vi "ROI_to_bbox.vi"(8 "Image path":path=path "C:/Users/Naomi Tan/Documents/Gillette/ML/STIR_ML_dev/LabView/original_images/IMG_6155.JPG", 9 "Bounding box size":dbl=300.0, 10 "ROI":T5, 11 "Image in":T1) -> (3 "bbox":T2)   [LabVIEW 2024]
uses:
  <vilib>/vision/Image Controls.llb/IMAQ Image.ctl
  controls/class.ctl
panel:
  out "Points":i32[](array[numeric])
  in  "Class Name:":T3 items=["nick", "hair", "cut"]
  out "Classes":string[][](array[string])
  in  "Init Classes":string[][](array[string])
  in  "Size":i32
  out "Bounding Boxes Out":T4(array[cluster])
  in  "Bounding Boxes In":T4(array[cluster])
  in  "Image In":T1
  out "Image Out":T1
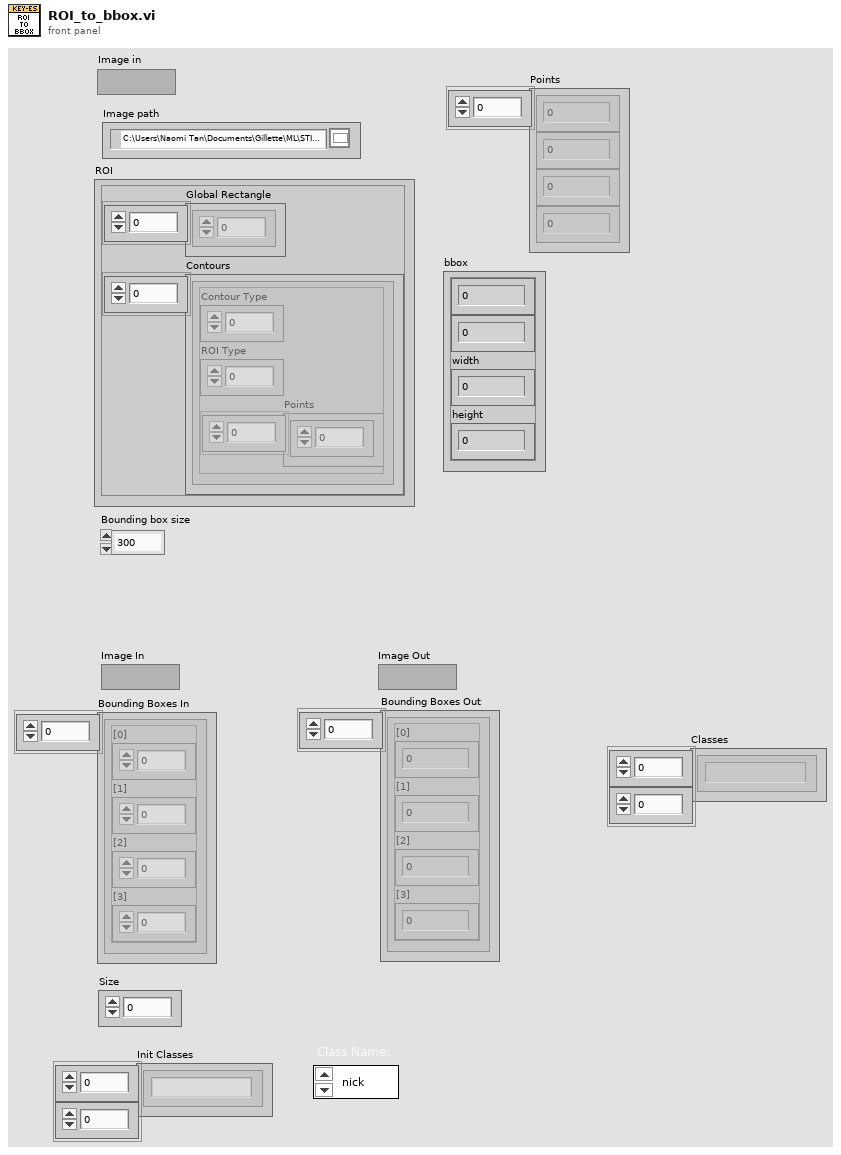
[diagram p1: front panel]
types:
  T1 = typedef "IMAQ Image.ctl" = refnum<image>
  T2 = cluster{"Numeric Control":dbl, "Numeric Control":dbl, "width":dbl, "height":dbl}
  T3 = typedef "Class.ctl" = u16
  T4 = cluster{"[0]":i32, "[1]":i32, "[2]":i32, "[3]":i32}[]
  T5 = cluster{"Global Rectangle":i32[], "Contours":cluster{"Contour Type":u32, "ROI Type":u32, "Points":i32[]}[]}
  T6 = cluster{"Contour Type":u32, "ROI Type":u32, "Points":i32[]}[]
  T7 = cluster{"Contour Type":u32, "ROI Type":u32, "Points":i32[]}
  T8 = typedef "imagedata.ctl" = cluster{"image type":i32, "image depth":i32, "image":u8[], "mask":u8[], "colors":u32[], "Rectangle":cluster{"left":i16, "top":i16, "right":i16, "bottom":i16}}
  T9 = cluster{dbl, dbl, "X Resolution":dbl, "Y Resolution":dbl}
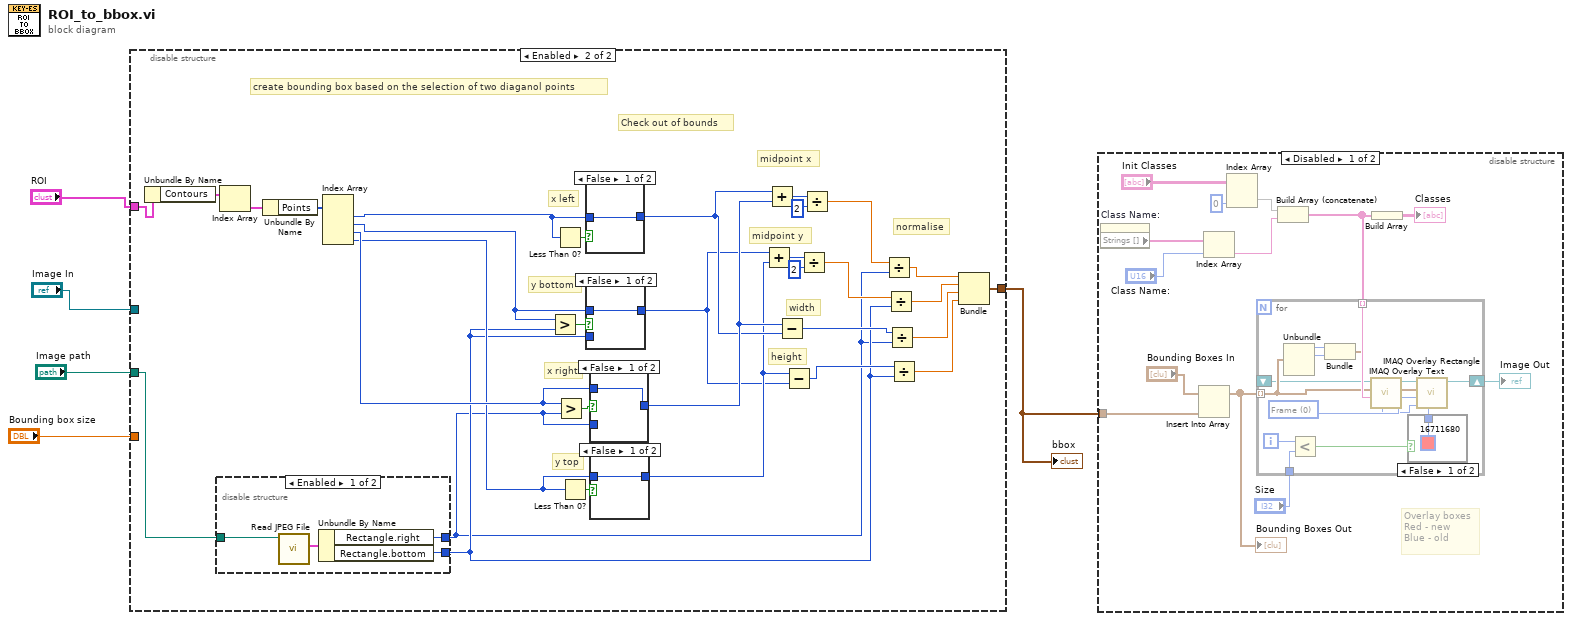
[diagram p0: block diagram]
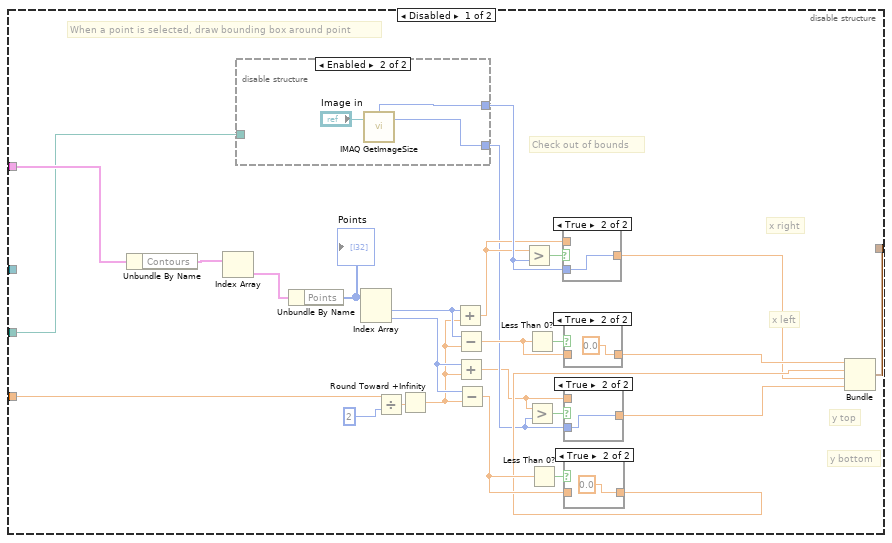
[diagram p2: hidden frame]
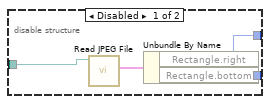
[diagram p3: hidden frame]
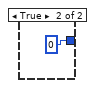
[diagram p8: hidden frame]
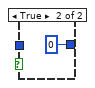
[diagram p11: hidden frame]
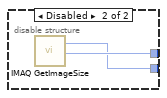
[diagram p12: hidden frame]
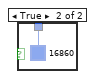
[diagram p13: hidden frame]
diagram:
  n1 = disable-structure shown="Enabled" {
    disable-tunnel: "ROI" -> [w9 w74]
    disable-tunnel: [w8 w71] -> w5
    disable-tunnel: "Bounding box size" -> [w7 _]
    disable-tunnel: "Image In" -> [_ _]
    disable-tunnel: "Image path" -> [w6 w69]
    frame Disabled {
      # "y bottom"
      # "y top"
      # "x left"
      # "x right"
      # "Check out of bounds"
      # "When a point is selected, draw bounding box around point"
      n2 = Unbundle By Name(w9) -> ("Contours"=w31:T6)
      n3 = Index Array(array=w31) -> (element=w30:T7)  [unwired: 1 in]
      n4 = disable-structure shown="Enabled" {
        disable-tunnel: [w34 w38] -> w16
        disable-tunnel: [w33 w37] -> w12
        disable-tunnel: w6 -> [w32 _]
        frame Disabled {
          n5 = call <vilib>:"Read JPEG File.vi"("path to JPEG file"=w32) -> ("image data"=w35:T8)  [unwired: 8 in, 2 out]
          n6 = Unbundle By Name(w35) -> ("Rectangle.right"=w34:i16, "Rectangle.bottom"=w33:i16)
        }
        frame Enabled {
          n7 = call "IMAQ GetImageSize"("Image"="Image in") -> ("Y Resolution"=w37:i32, "X Resolution"=w38:i32)  [unwired: 3 in, 1 out]
        }
      }
      n8 = Unbundle By Name(w30) -> ("Points"=w29:i32[])
      "Points" <- w29
      n9 = Index Array(array=w29) -> (element #1=w27:i32, element #2=w28:i32)  [unwired: 2 in]
      n10 = Divide(x=w7, y=2) -> (x/y=w25:dbl)
      n11 = Round Toward +Infinity(x=w25) -> (ceil(x): smallest int >= x=w24:dbl)
      n12 = Add(x=w27, y=w24) -> (x+y=w15:dbl)
      n13 = Subtract(x=w27, y=w24) -> (x-y=w22:dbl)
      n14 = Add(x=w28, y=w24) -> (x+y=w11:dbl)
      n15 = Subtract(x=w28, y=w24) -> (x-y=w19:dbl)
      n16 = Greater?(x=w15, y=w16) -> (0:w17:bool)
      n17 = Less Than 0?(x=w22) -> (x < 0?=w23:bool)
      n18 = Greater?(x=w11, y=w12) -> (0:w13:bool)
      n19 = Less Than 0?(x=w19) -> (x < 0?=w20:bool)
      n20 = case shown="True" w17 {
        tunnel: w16 -> [_ w46]
        tunnel: [w45 w46] -> w14
        tunnel: w15 -> [w45 _]
        frame False {
        }
        frame True {
        }
      }
      n21 = case shown="True" w23 {
        tunnel: w22 -> [w41 _]
        tunnel: [w41 0.0] -> w21
        frame False {
        }
        frame True {
        }
      }
      n22 = case shown="True" w13 {
        tunnel: [w43 w44] -> w10
        tunnel: w12 -> [_ w44]
        tunnel: w11 -> [w43 _]
        frame False {
        }
        frame True {
        }
      }
      n23 = case shown="True" w20 {
        tunnel: w19 -> [w39 _]
        tunnel: [w39 0.0] -> w18
        frame False {
        }
        frame True {
        }
      }
      n24 = Bundle(w21, w18, "X Resolution"=w14, "Y Resolution"=w10) -> (w8:T9)  [unwired: 1 in]
    }
    frame Enabled {
      # "normalise"
      # "height"
      # "width"
      # "midpoint y"
      # "midpoint x"
      # "y top"
      # "x right"
      # "y bottom"
      # "x left"
      # "Check out of bounds"
      # "create bounding box based on the selection of two diaganol points"
      n25 = Unbundle By Name(w74) -> ("Contours"=w78:T6)
      n26 = disable-structure shown="Enabled" {
        disable-tunnel: [w89 w92] -> w47
        disable-tunnel: [w88 w91] -> w48
        disable-tunnel: w69 -> [w87 _]
        frame Enabled {
          n27 = call <vilib>:"Read JPEG File.vi"("path to JPEG file"=w87) -> ("image data"=w90:T8)  [unwired: 8 in, 2 out]
          n28 = Unbundle By Name(w90) -> ("Rectangle.right"=w89:i16, "Rectangle.bottom"=w88:i16)
        }
        frame Disabled {
          n29 = call "IMAQ GetImageSize"() -> ("Y Resolution"=w91:i32, "X Resolution"=w92:i32)  [unwired: 4 in, 1 out]
        }
      }
      n30 = Index Array(array=w78) -> (element=w77:T7)  [unwired: 1 in]
      n31 = Unbundle By Name(w77) -> ("Points"=w76:i32[])
      n32 = Index Array(array=w76) -> (element #1=w68:i32, element #2=w75:i32, element #3=w70:i32, element #4=w66:i32)  [unwired: 4 in]
      n33 = Greater?(x=w75, y=w48) -> (0:w73:bool)
      n34 = Less Than 0?(x=w68) -> (x < 0?=w67:bool)
      n35 = Greater?(x=w70, y=w47) -> (0:w72:bool)
      n36 = Less Than 0?(x=w66) -> (x < 0?=w65:bool)
      n37 = case shown="False" w67 {
        tunnel: [w85 0 ("Numeric Control")] -> w59
        tunnel: w68 -> [w85 _]
        frame False {
        }
        frame True {
        }
      }
      n38 = case shown="False" w73 {
        tunnel: [w83 w84] -> w57
        tunnel: w75 -> [w83 _]
        tunnel: w48 -> [_ w84]
        frame False {
        }
        frame True {
        }
      }
      n39 = case shown="False" w72 {
        tunnel: [w81 w82] -> w60
        tunnel: w70 -> [w81 _]
        tunnel: w47 -> [_ w82]
        frame False {
        }
        frame True {
        }
      }
      n40 = case shown="False" w65 {
        tunnel: [w79 0 ("Numeric Control")] -> w58
        tunnel: w66 -> [w79 _]
        frame False {
        }
        frame True {
        }
      }
      n41 = Add(x=w57, y=w58) -> (x+y=w62:i32)
      n42 = Add(x=w59, y=w60) -> (x+y=w64:i32)
      n43 = Subtract(x=w60, y=w59) -> (x-y=w49:i32)
      n44 = Subtract(x=w58, y=w57) -> (x-y=w55:i32)
      n45 = Divide(x=w62, y=2) -> (x/y=w50:dbl)
      n46 = Divide(x=w64, y=2) -> (x/y=w56:dbl)
      n47 = Divide(x=w56, y=w47) -> (x/y=w54:dbl)
      n48 = Divide(x=w50, y=w48) -> (x/y=w53:dbl)
      n49 = Divide(x=w49, y=w47) -> (x/y=w52:dbl)
      n50 = Divide(x=w55, y=w48) -> (x/y=w51:dbl)
      n51 = Bundle(w54, w53, w52, w51) -> (w71:cluster{dbl, dbl, dbl, dbl})  [unwired: 1 in]
    }
  }
  "bbox" <- w5
  n52 = disable-structure shown="Disabled" {
    disable-tunnel: w5 -> [w106 _]
    frame Disabled {
      # "Overlay boxes\nRed - new\nBlue - old"
      n53 = property on="Class Name:" class="Ring (strict)"() -> ("Strings []"=w93:string[])  [unwired: 2 in, 2 out]
      n54 = Insert Into Array(array="Bounding Boxes In", new element=w106) -> (w104:T4)  [unwired: 1 in]
      "Bounding Boxes Out" <- w104
      n55 = Index Array(array=w93, index="Class Name:") -> (element=w99:string)
      n56 = Index Array(array="Init Classes", index (col)=0 ("disabled index (col)")) -> (element=w97:string[])  [unwired: 1 in]
      n57 = Build Array (concatenate)(w97, w99) -> (w100:string[])
      n58 = for {
        shift-right: [w119] -> w105
        shift-left: [w110] -> w103
        tunnel: w104 -> [w113] mode=indexing
        tunnel: "Size" -> [w115]
        tunnel: w100 -> [w114] mode=indexing
        i -> [w117]
        w118 = u32 0 items=["Frame", "Fill"] ("Drawing Mode (Frame)")
        n59 = Unbundle(w113) -> ("[0]"=w112:i32, "[1]"=w111:i32)  [unwired: 2 out]
        n60 = Less?(x=w117, y=w115) -> (x < y?=w116:bool)
        n61 = Bundle("[0]"=w112, "[1]"=w111) -> (w108:cluster{"[0]":i32, "[1]":i32})  [unwired: 1 in]
        n62 = case shown="False" w116 {
          tunnel: [u32 16711680 ("Color") u32 16860 ("Color")] -> w107
          frame False {
          }
          frame True {
          }
        }
        n63 = call "IMAQ Overlay Text"("Text Color (black)"=w107, "String"=w114, "Origin"=w108, "Image"=w110) -> ("Image Out"=w109:T1)  [unwired: 6 in, 1 out]
        n64 = call "IMAQ Overlay Rectangle"("Color"=w107, "Drawing Mode (Frame)"=w118, "Rectangle"=w113, "Image"=w109) -> ("Image Out"=w119:T1)  [unwired: 6 in, 1 out]
      }
      "Image Out" <- w105
      n65 = Build Array(w100) -> (→"Classes":string[][])
    }
    frame Enabled {
    }
  }
